vi "SerialDataReadWrite_3CH_parallel.vi"() -> ()   [LabVIEW 2024]
uses:
  <vilib>/Instr/_visa.llb/VISA Configure Serial Port (Instr).vi
  <vilib>/Utility/file.llb/Write Delimited Spreadsheet (DBL).vi
panel:
  in  "VISA resource name":refnum<visa-resource-name>="COM8"
  out "Waveform Chart":sgl[][](graph)
  in  "file path":path=path "C:/temp/test1.txt"
  out "error out":errorcluster
  out "dt (ms)":u32
  out "freq (hz)":dbl
  out "Number of Bytes at Serial Port":u32
  out "byte read count":u32
  in  "stop":bool
  out "read buffer":string
  # "NB: record data until STOP is pressed"
  # "MAKE SURE TO ADD FILE TO THE LAB3 FOLDER UNEDR STUDIES"
  # "Add a file name!"
  # "STOP BUTTON USES ANOTHER MECHANICAL ACTION"
  # "Select!"
  # "Wafeform chart is a bit janky with unexpected resets"
  # "<- READ THE LOOP FREQUENCY HERE"
  # "The Dequeue Element error"
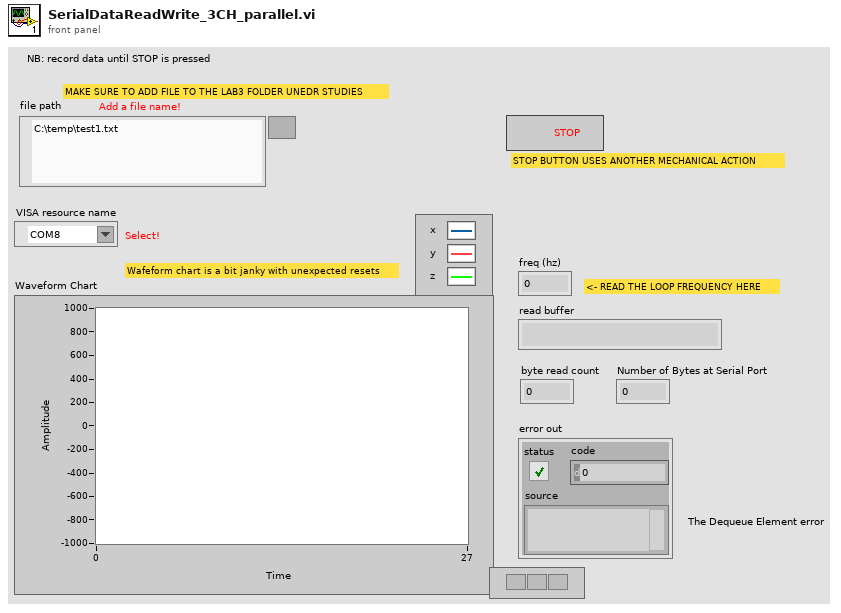
[diagram p1: front panel]
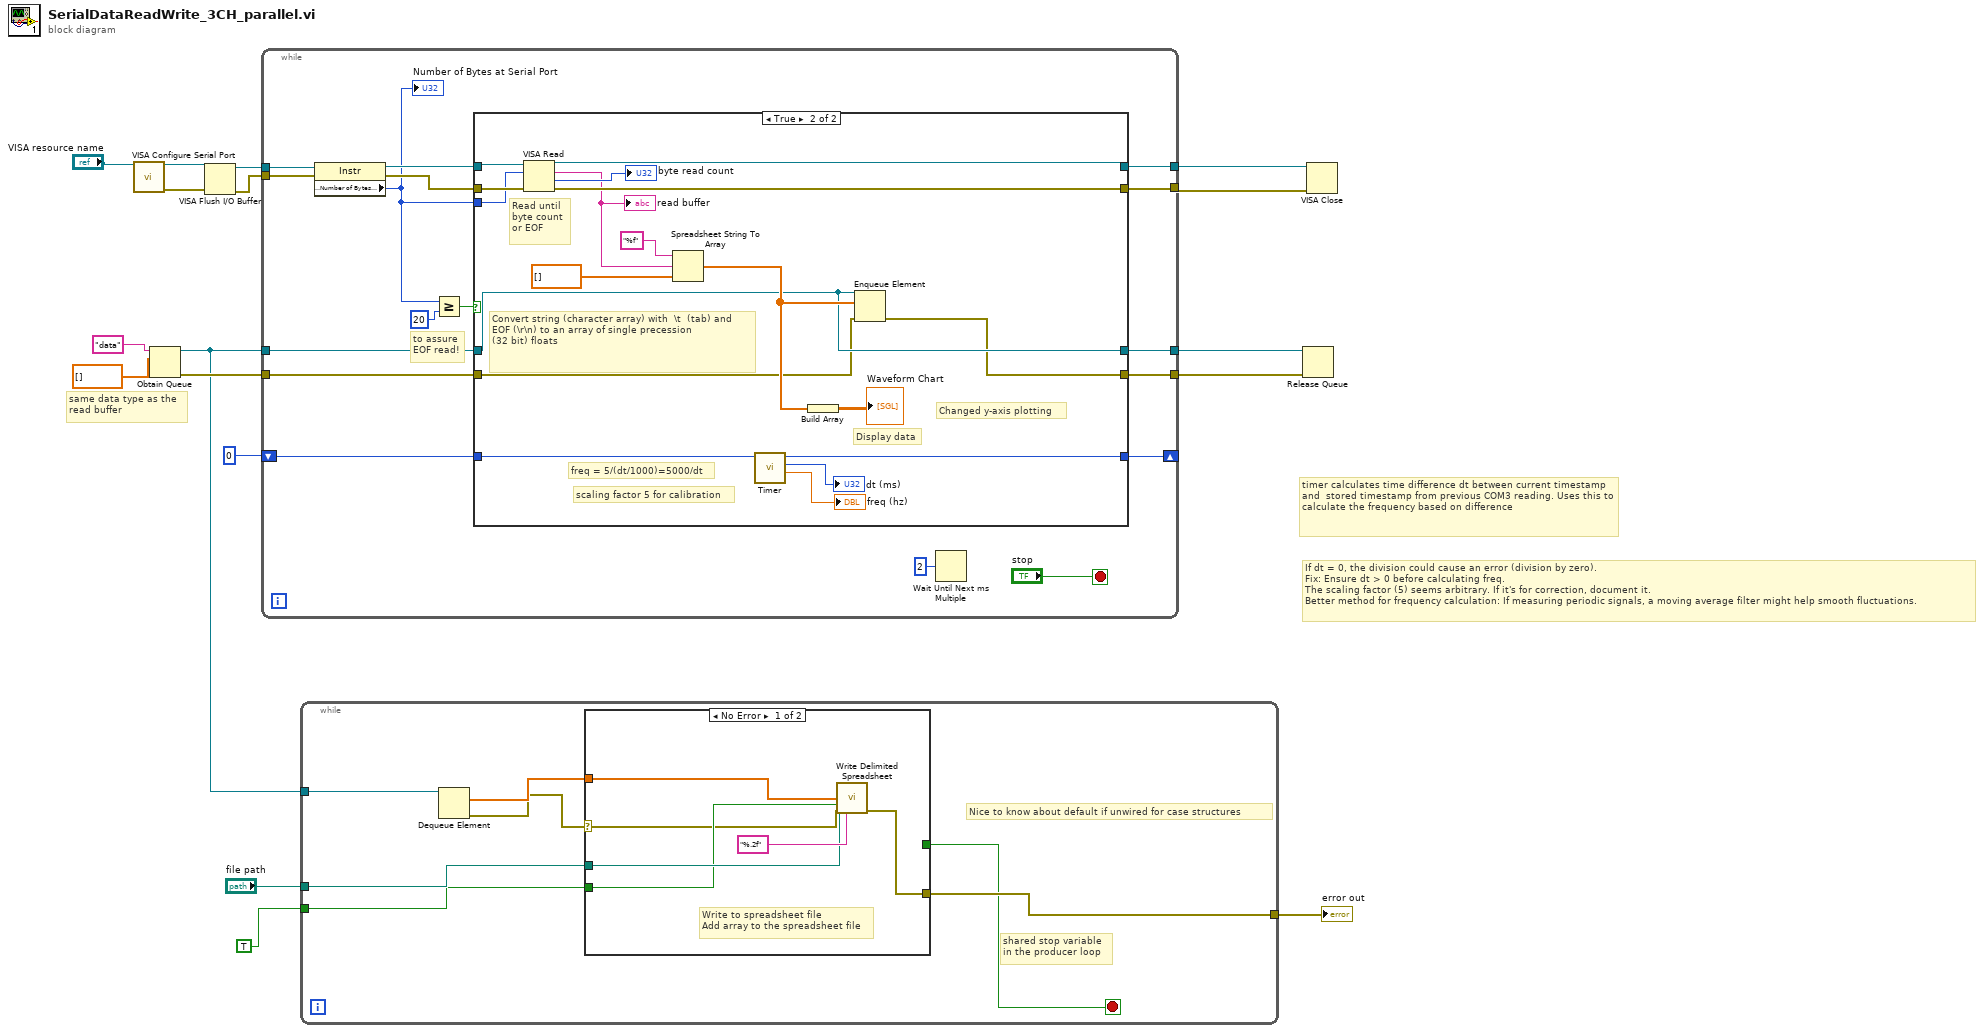
[diagram p0: block diagram]
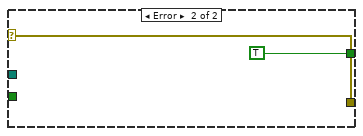
[diagram p2: hidden frame]
diagram:
  # "timer calculates time difference dt between current timestamp and  stored timestamp from previous COM3 reading. Uses this to calculate the frequency based on difference"
  # "If dt = 0, the division could cause an error (division by zero).\nFix: Ensure dt > 0 before calculating freq.\nThe scaling factor (5) seems arbitrary. If it's for correction, document it.\nBetter method for frequency calculation: If measuring periodic signals, a moving average filter might help smooth fluctuations."
  # "same data type as the \nread buffer"
  n1 = call-poly "VISA Configure Serial Port"("VISA resource name"="VISA resource name") -> ("VISA resource name out"=w14:refnum<visa-resource-name>, "error out"=w13:errorcluster)  [unwired: 13 in]
  n2 = Obtain Queue(name (unnamed)="data", element data type=sgl[] [] ("array type (2D Dbl)")) -> (queue out=w4:refnum<queue>, error out=w5:errorcluster)  [unwired: 3 in, 1 out]
  n3 = VISA Flush I/O Buffer(VISA resource name=w14, error in (no error)=w13) -> (VISA resource name out=w12:refnum<visa-resource-name>, error out=w11:errorcluster)  [unwired: 1 in]
  n4 = while {
    tunnel: w12 -> [w34]
    tunnel: w11 -> [w33]
    tunnel: [w30] -> w16
    tunnel: [w29] -> w15
    shift-right: [w22] -> _
    shift-left: u32 0 -> [w23]
    tunnel: w4 -> [w21]
    tunnel: [w20] -> w7
    tunnel: [w19] -> w6
    tunnel: w5 -> [w18]
    stop <- "stop" stop-if-true
    # "to assure\nEOF read!"
    n5 = property class="Instr"(reference=w34, error in=w33) -> (reference out=w31:refnum<visa-resource-name>, error out=w32:errorcluster, "Serial Settings:Number of Bytes at Serial Port"=w25:u32)
    "Number of Bytes at Serial Port" <- w25
    n6 = Greater Or Equal?(x=w25, y=u32 20) -> (x >= y?=w26:bool)
    n7 = case shown="True" w26 {
      tunnel: w32 -> [w38 w57]
      tunnel: w31 -> [w39 w56]
      tunnel: w25 -> [_ w55]
      tunnel: [w39 w54] -> w30
      tunnel: [w38 w53] -> w29
      tunnel: w23 -> [w37 w51]
      tunnel: [w37 w50] -> w22
      tunnel: w21 -> [w35 w43]
      tunnel: [w35 w43] -> w20
      tunnel: [w36 w42] -> w19
      tunnel: w18 -> [w36 w41]
      frame False {
      }
      frame True {
        # "scaling factor 5 for calibration"
        # "freq = 5/(dt/1000)=5000/dt"
        # "Changed y-axis plotting"
        # "Display data"
        # "Convert string (character array) with  \\t  (tab) and \nEOF (\\r\\n) to an array of single precession \n(32 bit) floats"
        # "Read until\nbyte count\nor EOF"
        n8 = VISA Read(VISA resource name=w56, byte count=w55, error in (no error)=w57) -> (VISA resource name out=w54:refnum<visa-resource-name>, read buffer=w40:string, return count=→"byte read count":u32, error out=w53:errorcluster)
        "read buffer" <- w40
        n9 = Spreadsheet String To Array(format string="%f", spreadsheet string=w40, array type (2D Dbl)=sgl[] []) -> (array=w44:sgl[])  [unwired: 1 in]
        n10 = call "Timer.vi"("Previous_ms"=w51) -> ("freq (hz)"=→"freq (hz)":dbl, "dt (ms)"=→"dt (ms)":u32, "Next_ms"=w50:u32)  [unwired: 8 in]
        n11 = Build Array(w44) -> (→"Waveform Chart":sgl[][])
        n12 = Enqueue Element(queue=w43, element=w44, error in (no error)=w41) -> (error out=w42:errorcluster)  [unwired: 1 in, 2 out]
      }
    }
    n13 = Wait Until Next ms Multiple(millisecond multiple=u32 2) -> ()  [unwired: 1 out]
  }
  n14 = while {
    tunnel: w4 -> [w64]
    tunnel: "file path" -> [w62]
    tunnel: TRUE ("append to file? (new file:F)") -> [w61]
    tunnel: [w60] -> w1
    stop <- w59 stop-if-true
    # "Nice to know about default if unwired for case structures"
    # "shared stop variable \nin the producer loop"
    n15 = Dequeue Element(queue=w64) -> (element=w63:sgl[], error out=w58:errorcluster)  [unwired: 2 in, 2 out]
    n16 = case shown="No Error" w58 {
      selector: w58 -> [w65 w71]
      tunnel: w63 -> [w69 _]
      tunnel: w62 -> [w68 _]
      tunnel: w61 -> [w67 _]
      tunnel: [w66 w71] -> w60
      tunnel: [_ TRUE] -> w59
      frame No Error {
        # "Write to spreadsheet file\nAdd array to the spreadsheet file"
        n17 = call-poly <vilib>:"Write Delimited Spreadsheet.vi"("file path (dialog if empty)"=w68, "format (%.3f)"="%.2f", "1D data"=w69, "append to file? (new file:F)"=w67, "error in (no error)"=w65) -> ("error out"=w66:errorcluster)  [unwired: 9 in, 1 out]
      }
      frame Error {
      }
    }
  }
  "error out" <- w1
  n18 = Release Queue(queue=w7, error in (no error)=w6) -> ()  [unwired: 1 in, 3 out]
  n19 = VISA Close(VISA resource name=w16, error in (no error)=w15) -> ()  [unwired: 1 out]
